vi "告警码字段定义.vi"(11 "告警代码":u16) -> (1 "故障详情":string, 2 "通用告警信息":string, 3 "字符串":string)   [LabVIEW 2016, in "斯坦道总磷.lvlib"]
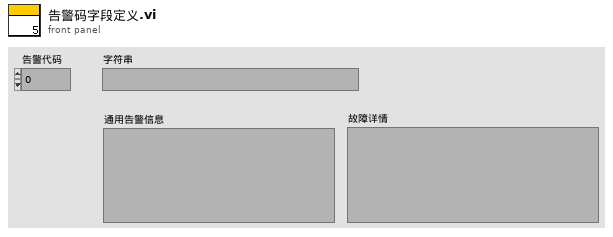
[diagram p1: front panel]
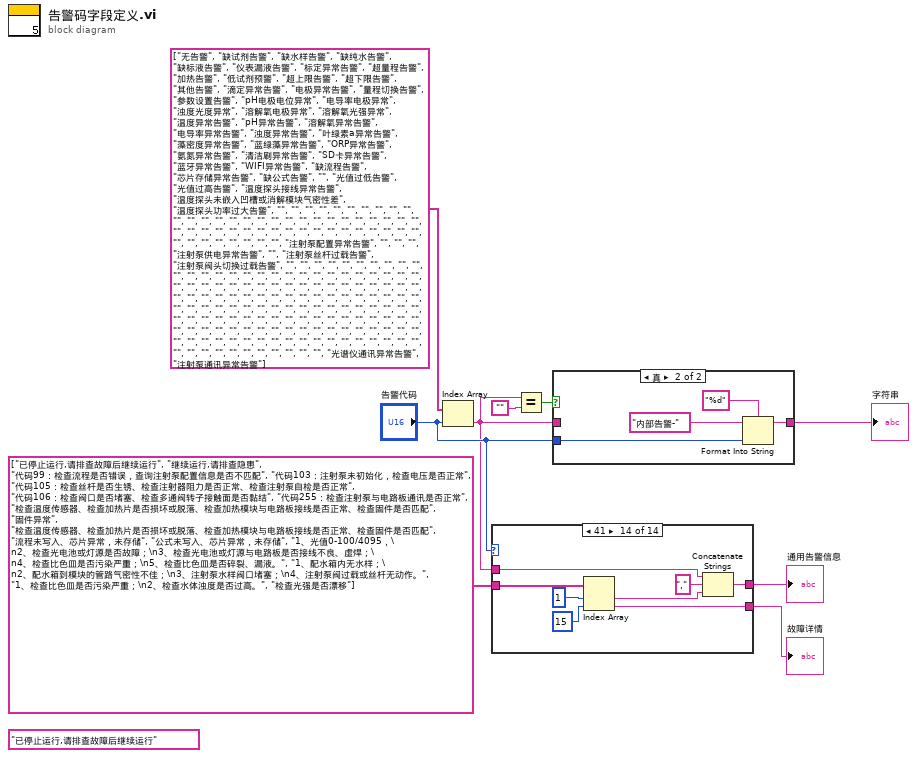
[diagram p0: block diagram]
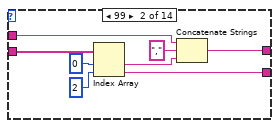
[diagram p3: hidden frame]
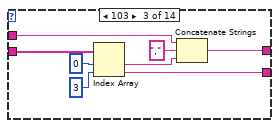
[diagram p4: hidden frame]
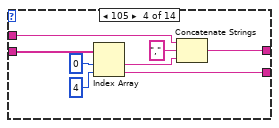
[diagram p5: hidden frame]
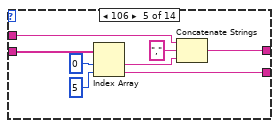
[diagram p6: hidden frame]
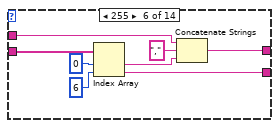
[diagram p7: hidden frame]
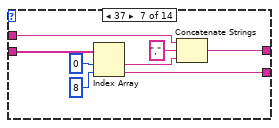
[diagram p8: hidden frame]
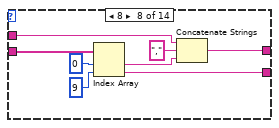
[diagram p9: hidden frame]
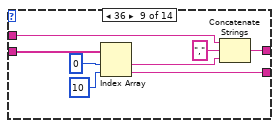
[diagram p10: hidden frame]
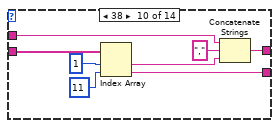
[diagram p11: hidden frame]
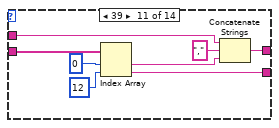
[diagram p12: hidden frame]
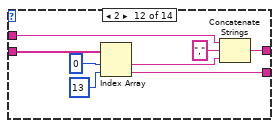
[diagram p13: hidden frame]
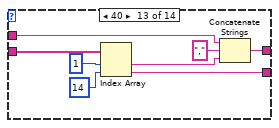
[diagram p14: hidden frame]
diagram:
  (unwired) "已停止运行,请排查故障后继续运行" ("工作状态")
  n1 = Index Array(array=string[] ["无告警", "缺试剂告警", "缺水样告警", "缺纯水告警", "缺标液告警", "仪表漏液告警", "标定异常告警", "超量程告警", "加热告警", "低试剂预警", "超上限告警", "超下限告警", "其他告警", "滴定异常告警", "电极异常告警", "量程切换告警", "参数设置告警", "pH电极电位异常", "电导率电极异常", "浊度光度异常", "溶解氧电极异常", "溶解氧光强异常", "温度异常告警", "pH异常告警", "溶解氧异常告警", "电导率异常告警", "浊度异常告警", "叶绿素a异常告警", "藻密度异常告警", "蓝绿藻异常告警", "ORP异常告警", "氨氮异常告警", "清洁刷异常告警", "SD卡异常告警", "蓝牙异常告警", "WIFI异常告警", "缺流程告警", "芯片存储异常告警", "缺公式告警", "", "光值过低告警", "光值过高告警", "温度探头接线异常告警", "温度探头未嵌入凹槽或消解模块气密性差", "温度探头功率过大告警", "", "", "", "", "", "", "", "", "", "", "", "", "", "", "", "", "", "", "", "", "", "", "", "", "", "", "", "", "", "", "", "", "", "", "", "", "", "", "", "", "", "", "", "", "", "", "", "", "", "", "", "", "", "", "注射泵配置异常告警", "", "", "", "注射泵供电异常告警", "", "注射泵丝杆过载告警", "注射泵阀头切换过载告警", "", "", "", "", "", "", "", "", "", "", "", "", "", "", "", "", "", "", "", "", "", "", "", "", "", "", "", "", "", "", "", "", "", "", "", "", "", "", "", "", "", "", "", "", "", "", "", "", "", "", "", "", "", "", "", "", "", "", "", "", "", "", "", "", "", "", "", "", "", "", "", "", "", "", "", "", "", "", "", "", "", "", "", "", "", "", "", "", "", "", "", "", "", "", "", "", "", "", "", "", "", "", "", "", "", "", "", "", "", "", "", "", "", "", "", "", "", "", "", "", "", "", "", "", "", "", "", "", "", "", "", "", "", "", "", "", "", "", "", "", "", "", "", "", "", "", "", "光谱仪通讯异常告警", "注射泵通讯异常告警"], index="告警代码") -> (element=w1:string)
  n2 = case shown="41" "告警代码" {
    tunnel: string[] ["已停止运行,请排查故障后继续运行", "继续运行,请排查隐患", "代码99：检查流程是否错误，查询注射泵配置信息是否不匹配", "代码103：注射泵未初始化，检查电压是否正常", "代码105：检查丝杆是否生锈、检查注射器阻力是否正常、检查注射泵自检是否正常", "代码106：检查阀口是否堵塞、检查多通阀转子接触面是否黏结", "代码255：检查注射泵与电路板通讯是否正常", "检查温度传感器、检查加热片是否损坏或脱落、检查加热模块与电路板接线是否正常、检查固件是否匹配", "固件异常", "检查温度传感器、检查加热片是否损坏或脱落、检查加热模块与电路板接线是否正常、检查固件是否匹配", "流程未写入、芯片异常，未存储", "公式未写入、芯片异常，未存储", "1、光值0-100/4095，\n2、检查光电池或灯源是否故障；\n3、检查光电池或灯源与电路板是否接线不良、虚焊；\n4、检查比色皿是否污染严重；\n5、检查比色皿是否碎裂、漏液。", "1、配水箱内无水样；\n2、配水箱到模块的管路气密性不佳；\n3、注射泵水样阀口堵塞；\n4、注射泵阀过载或丝杆无动作。", "1、检查比色皿是否污染严重；\n2、检查水体浊度是否过高。", "检查光强是否漂移"] -> [_ w18 w26 w34 w42 w50 w58 w66 w74 w82 w90 w98 w106 w114]
    tunnel: [w10 w13 w21 w29 w37 w45 w53 w61 w69 w77 w85 w93 w101 w109] -> w3
    tunnel: [_ w14 w22 w30 w38 w46 w54 w62 w70 w78 w86 w94 w102 w110] -> w2
    tunnel: w1 -> [w10 w12 w20 w28 w36 w44 w52 w60 w68 w76 w84 w92 w100 w108]
    frame 0, Default {
    }
    frame 99 {
      n3 = Index Array(array=w18, index #1=0 ("索引"), index #2=2 ("索引")) -> (element #1=w16:string, element #2=w14:string)
      n4 = Concatenate Strings(w12, "," ("字符串"), w16) -> (w13:string)
    }
    frame 103 {
      n5 = Index Array(array=w26, index #1=0 ("索引"), index #2=3 ("索引")) -> (element #1=w24:string, element #2=w22:string)
      n6 = Concatenate Strings(w20, "," ("字符串"), w24) -> (w21:string)
    }
    frame 105 {
      n7 = Index Array(array=w34, index #1=0 ("索引"), index #2=4 ("索引")) -> (element #1=w32:string, element #2=w30:string)
      n8 = Concatenate Strings(w28, "," ("字符串"), w32) -> (w29:string)
    }
    frame 106 {
      n9 = Index Array(array=w42, index #1=0 ("索引"), index #2=5 ("索引")) -> (element #1=w40:string, element #2=w38:string)
      n10 = Concatenate Strings(w36, "," ("字符串"), w40) -> (w37:string)
    }
    frame 255 {
      n11 = Index Array(array=w50, index #1=0 ("索引"), index #2=6 ("索引")) -> (element #1=w48:string, element #2=w46:string)
      n12 = Concatenate Strings(w44, "," ("字符串"), w48) -> (w45:string)
    }
    frame 37 {
      n13 = Index Array(array=w58, index #1=0 ("索引"), index #2=8 ("索引")) -> (element #1=w56:string, element #2=w54:string)
      n14 = Concatenate Strings(w52, "," ("字符串"), w56) -> (w53:string)
    }
    frame 8 {
      n15 = Index Array(array=w66, index #1=0 ("索引"), index #2=9 ("索引")) -> (element #1=w64:string, element #2=w62:string)
      n16 = Concatenate Strings(w60, "," ("字符串"), w64) -> (w61:string)
    }
    frame 36 {
      n17 = Index Array(array=w74, index #1=0 ("索引"), index #2=10 ("索引")) -> (element #1=w72:string, element #2=w70:string)
      n18 = Concatenate Strings(w68, "," ("字符串"), w72) -> (w69:string)
    }
    frame 38 {
      n19 = Index Array(array=w82, index #1=1 ("索引"), index #2=11 ("索引")) -> (element #1=w80:string, element #2=w78:string)
      n20 = Concatenate Strings(w76, "," ("字符串"), w80) -> (w77:string)
    }
    frame 39 {
      n21 = Index Array(array=w90, index #1=0 ("索引"), index #2=12 ("索引")) -> (element #1=w88:string, element #2=w86:string)
      n22 = Concatenate Strings(w84, "," ("字符串"), w88) -> (w85:string)
    }
    frame 2 {
      n23 = Index Array(array=w98, index #1=0 ("索引"), index #2=13 ("索引")) -> (element #1=w96:string, element #2=w94:string)
      n24 = Concatenate Strings(w92, "," ("字符串"), w96) -> (w93:string)
    }
    frame 40 {
      n25 = Index Array(array=w106, index #1=1 ("索引"), index #2=14 ("索引")) -> (element #1=w104:string, element #2=w102:string)
      n26 = Concatenate Strings(w100, "," ("字符串"), w104) -> (w101:string)
    }
    frame 41 {
      n27 = Index Array(array=w114, index #1=1 ("索引"), index #2=15 ("索引")) -> (element #1=w112:string, element #2=w110:string)
      n28 = Concatenate Strings(w108, "," ("字符串"), w112) -> (w109:string)
    }
  }
  "通用告警信息" <- w3
  "故障详情" <- w2
  n29 = Equal?(x=w1, y="") -> (x = y?=w7:bool)
  n30 = case shown="真" w7 {
    tunnel: [w115 w117] -> w6
    tunnel: w1 -> [w115 _]
    tunnel: "告警代码" -> [_ w116]
    frame False {
    }
    frame True {
      n31 = Format Into String(format string="%d" ("格式字符串"), initial string="内部告警-" ("工作状态"), w116) -> (resulting string=w117:string)  [unwired: 1 in, 1 out]
    }
  }
  "字符串" <- w6
